vi "flexray enable frame.vi"(8 "error in (no error)":errorcluster caption="错误输入（无错误）", 10 "FR_Frame":T1, 11 "path in":path) -> (0 "error out":errorcluster caption="错误输出", 2 "function return":i32, 3 "path out":path)   [LabVIEW 2014]
doc: "TSAPI(s32)flexray_enable_frame(const s32 AChnIdx,const u8 ASlot,const u8 ABaseCycle,const u8 ACycleRep,const s32 ATimeoutMs);"
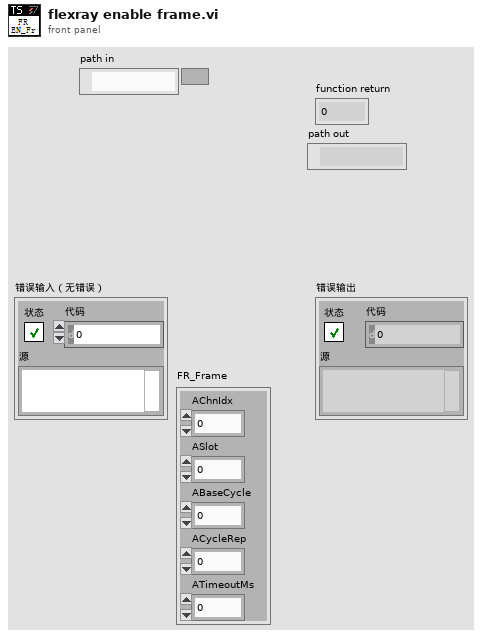
[diagram p1: front panel]
types:
  T1 = cluster{"AChnIdx":i32, "ASlot":u8, "ABaseCycle":u8, "ACycleRep":u8, "ATimeoutMs":i32}
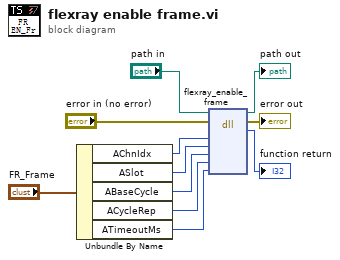
[diagram p0: block diagram]
diagram:
  n1 = Unbundle By Name("FR_Frame") -> ("AChnIdx"=w5:i32, "ASlot"=w4:u8, "ABaseCycle"=w3:u8, "ACycleRep"=w2:u8, "ATimeoutMs"=w1:i32)
  n2 = dll-call lib="D:/Work/LabVIEW Code/TSMaster Labview SDK/LabVIEW/LabVIEW-TSMasterAPI_CLN/TSMasterAPI_LabVIEW-2024-10-08 14-20-13/Not_organized_vi/TSMaster.*" fn="flexray_enable_frame"(path in="path in", error in="error in (no error)", "AChnIdx"=w5, "ASlot"=w4, "ABaseCycle"=w3, "ACycleRep"=w2, "ATimeoutMs"=w1) -> (path out=→"path out":path, error out=→"error out":errorcluster, "返回类型"=→"function return":i32)  [unwired: 6 in]
